vi "Disconnect.vi"(8 "error in":errorcluster, 11 "2575 in":refnum<class "2575.lvclass">) -> (0 "error out":errorcluster, 3 "2575 out":refnum<class "2575.lvclass">)   [LabVIEW 2019, in "2575.lvlib" / "2575.lvclass"]
doc: "Override VI, close communication with the instrument and cleanly destroy the resource reference."
uses:
  Library/2575.lvclass
  Library/2575.lvclass/2575.ctl
  Accessors/Read Local Resource.vi
  Accessors/Write Local Resource.vi
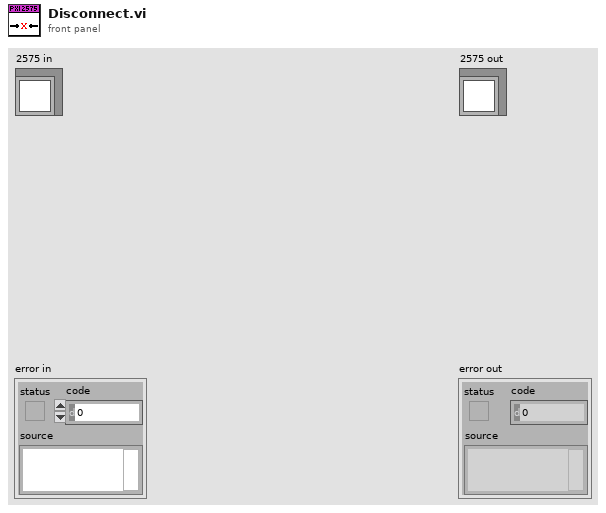
[diagram p1: front panel]
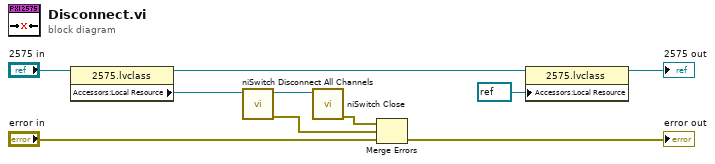
[diagram p0: block diagram]
diagram:
  n1 = property class="2575.lvclass"(reference="2575 in") -> (reference out=w4:refnum<class "2575.lvclass">, "Accessors:Local Resource"=w6:refnum<k15>)  [unwired: 1 in, 1 out]
  n2 = call <instrlib>:"niSwitch Disconnect All Channels.vi"("instrument handle"=w6) -> ("error out"=w1:errorcluster, "instrument handle out"=w2:refnum<k15>)  [unwired: 9 in]
  n3 = call <instrlib>:"niSwitch Close.vi"("instrument handle"=w2) -> ("error out"=w3:errorcluster)  [unwired: 10 in]
  n4 = Merge Errors(w3, w1, "error in") -> (→"error out":errorcluster)
  n5 = property class="2575.lvclass"(reference=w4, "Accessors:Local Resource"=refnum<k15> refnum ("Local Resource")) -> (reference out=→"2575 out":refnum<class "2575.lvclass">)  [unwired: 1 in, 1 out]
